vi "Graph with cursors Facade.vi"(0 "Data In":T4, 2 "Display State In":T2, 3 "Container State":T3) -> (6 "Data Out":T4, 7 "Display State Out":T2, 8 "Action":T1)   [LabVIEW 2014, in "Graph with cursors XControl.xctl"]
uses:
  Graph with cursors XControl.xctl
  Graph with cursors Data.ctl
  <vilib>/_xctls/Container State.ctl
  Graph with cursors State.ctl
  <vilib>/_xctls/Action.ctl
  <vilib>/_xctls/XControlSupport.lvlib
panel:
  in  "SaveCursors":bool
  in  "CursorPath":path
  in  "LoadCursors":bool
  in  "Prefix":string
  in  "Save":bool
  in  "Cursor pairs":u32=1 min=1
  out "Graph":waveform(dbl)(graph)
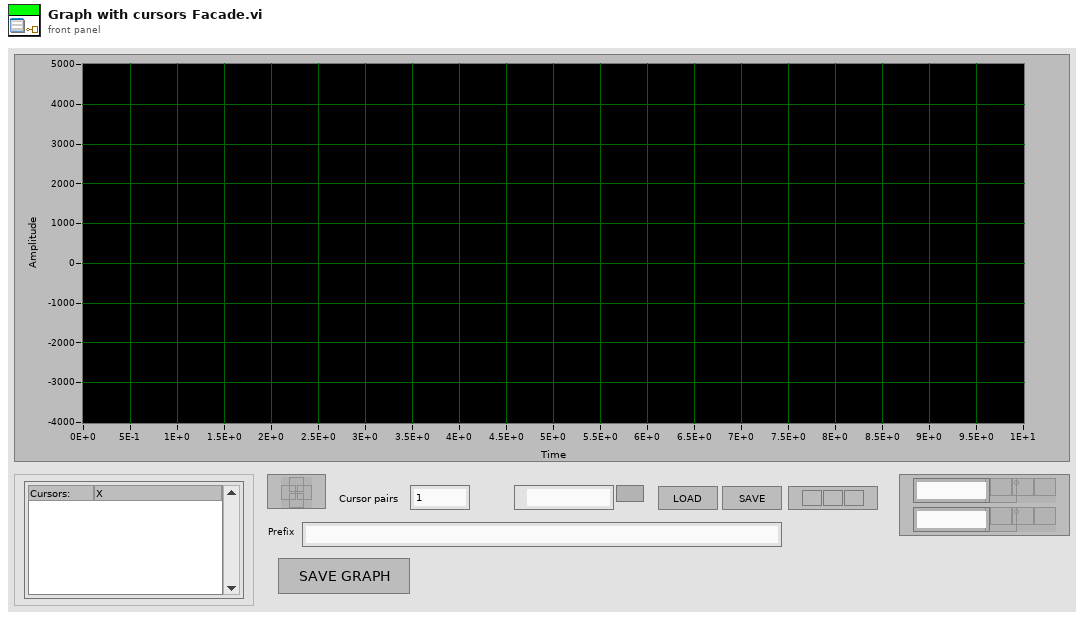
[diagram p1: front panel]
types:
  T1 = typedef "XControlSupport.lvlib/Action.ctl" = cluster{"Data Changed?":bool, "State Changed?":bool, "Action Name":string}
  T2 = typedef "Graph with cursors XControl.xctl/Graph with cursors State.ctl" = cluster{"Cursor names":string[], "Cursor positions":dbl[], "Cursor pairs":i32, "Graph":refnum<vi>, "Prefix":string, "Base path":path}
  T3 = typedef "XControlSupport.lvlib/Container State.ctl" = cluster{"Indicator?":bool, "Run Mode?":bool, " Refnum":refnum<vi>}
  T4 = typedef "Graph with cursors XControl.xctl/Graph with cursors Data.ctl" = waveform(dbl)
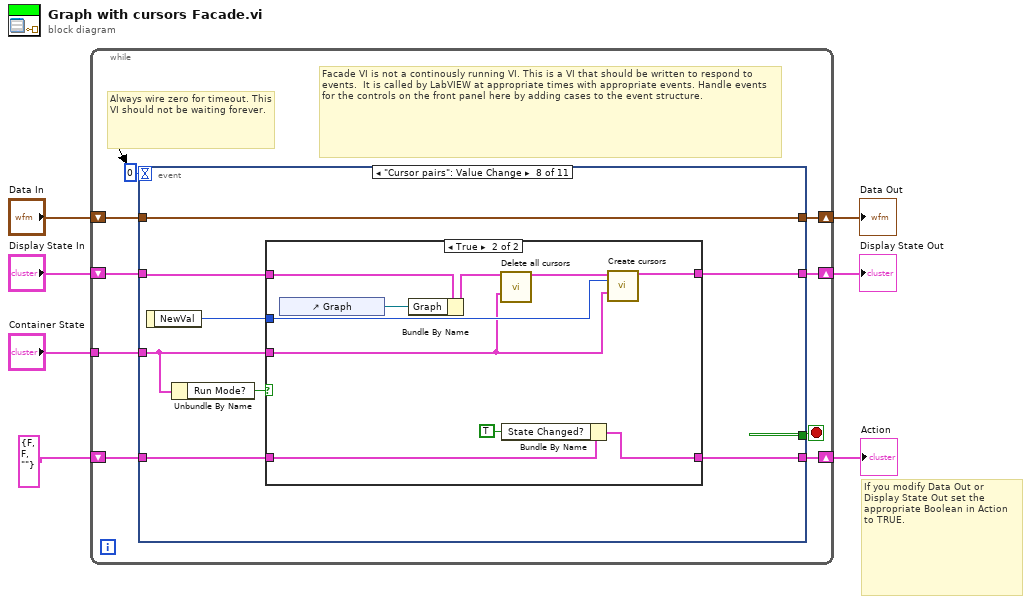
[diagram p0: block diagram]
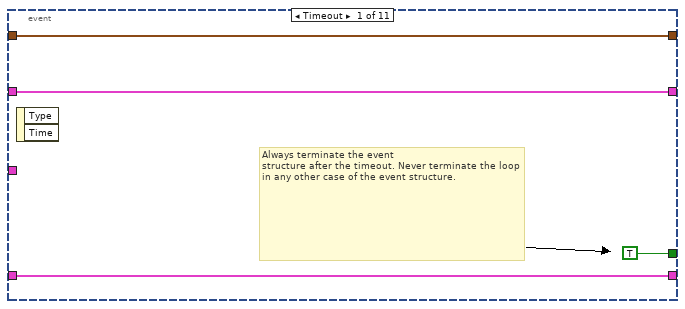
[diagram p2: hidden frame]
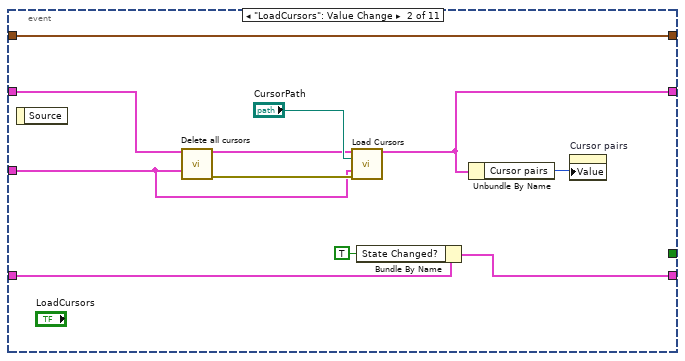
[diagram p3: hidden frame]
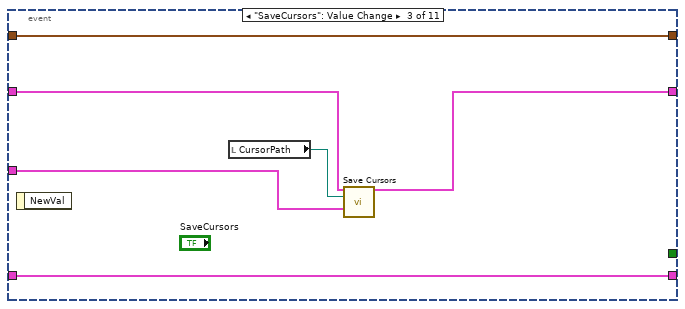
[diagram p4: hidden frame]
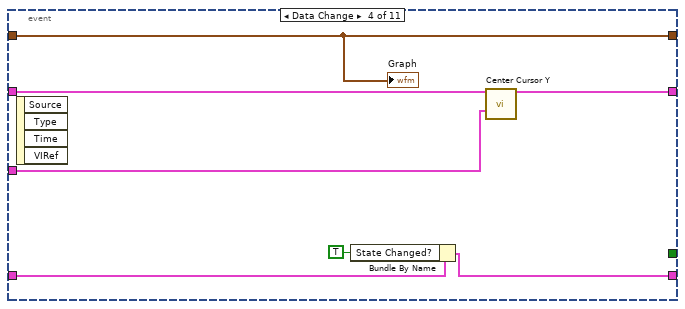
[diagram p5: hidden frame]
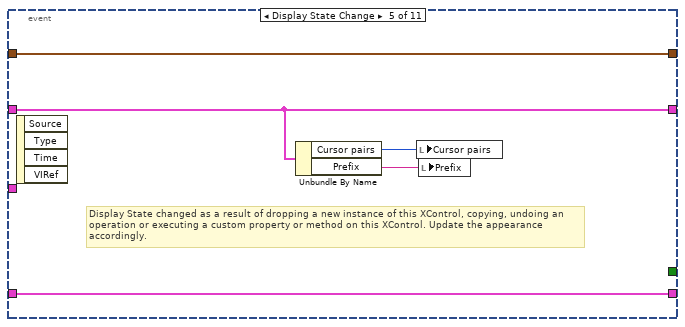
[diagram p6: hidden frame]
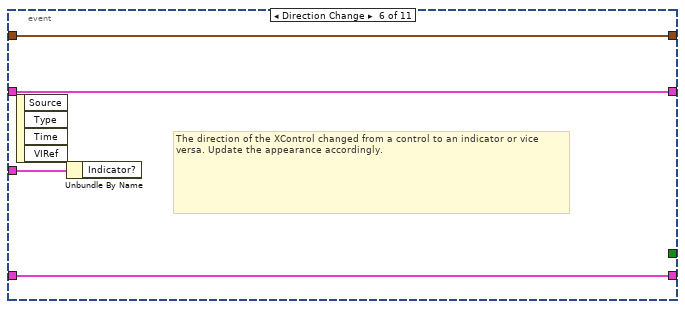
[diagram p7: hidden frame]
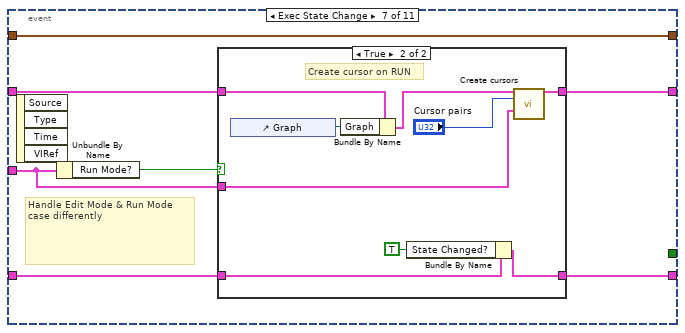
[diagram p8: hidden frame]
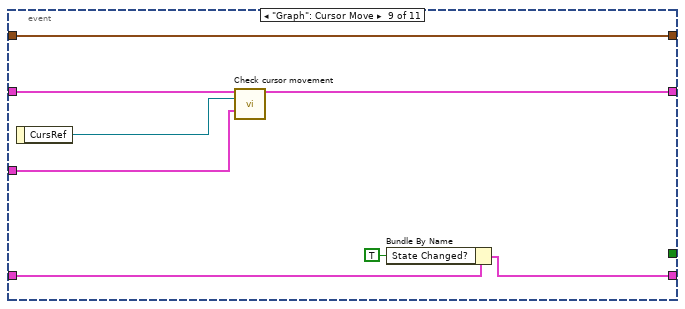
[diagram p11: hidden frame]
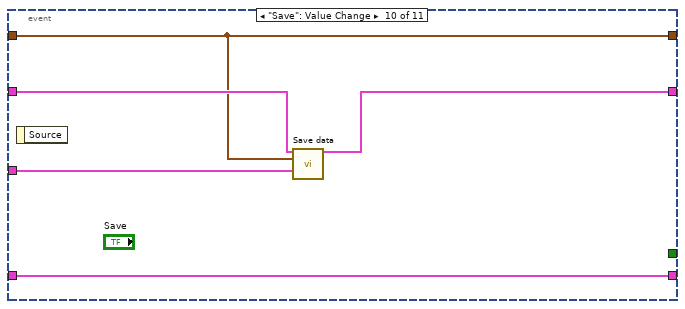
[diagram p12: hidden frame]
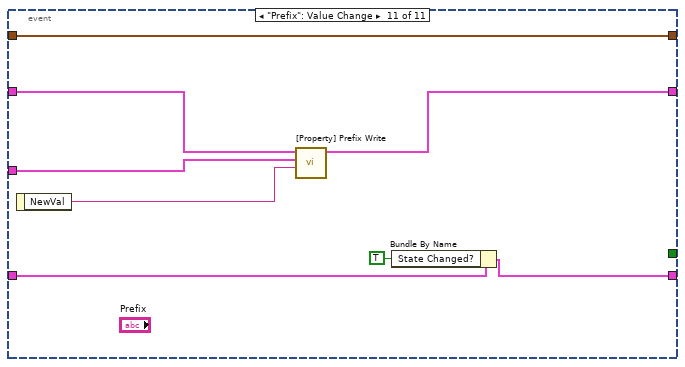
[diagram p13: hidden frame]
diagram:
  # "If you modify Data Out or\nDisplay State Out set the\nappropriate Boolean in Action\nto TRUE."
  n1 = while {
    shift-right: [w15] -> w4
    shift-left: "Display State In" -> [w16]
    tunnel: "Container State" -> [w12]
    shift-right: [w10] -> w7
    shift-left: "Data In" -> [w11]
    shift-right: [w8] -> w3
    shift-left: T1 {"Data Changed?"=FALSE, "State Changed?"=FALSE, "Action Name"=""} ("Action") -> [w9]
    stop <- w14 stop-if-true
    # "Facade VI is not a continously running VI. This is a VI that should be written to respond to events.  It is called by LabVIEW at appropriate times with appropriate events. Handle events for the controls on the front panel here by adding cases to the event structure."
    # "Always wire zero for timeout. This\nVI should not be waiting forever."
    n2 = event shown="[7] \"Cursor pairs\": Value Change" {
      selector: _ -> [_ _ _ _ _ _ _ _ _ _ _]
      dyn-events: _ -> [_ _ _ _ _ _ _ _ _ _ _]
      timeout: 0 -> [_ _ _ _ _ _ _ _ _ _ _]
      tunnel: w16 -> [w18 w23 w34 w42 w47 w52 w59 w76 w98 w103 w108]
      tunnel: [w18 w22 w33 w43 w47 w52 w57 w78 w97 w102 w107] -> w15
      tunnel: [TRUE _ _ _ _ _ _ _ _ _ _] -> w14
      tunnel: w12 -> [_ w24 w32 w38 _ w53 w54 w73 w96 w101 w106]
      tunnel: w11 -> [w17 w31 w37 w44 w49 w51 w60 w79 w99 w100 w112]
      tunnel: [w17 w31 w37 w44 w49 w51 w60 w79 w99 w100 w112] -> w10
      tunnel: [w19 w27 w36 w39 w48 w50 w56 w74 w94 w104 w110] -> w8
      tunnel: w9 -> [w19 w28 w36 w41 w48 w50 w55 w75 w93 w104 w111]
      event Timeout {
        # "Always terminate the event\nstructure after the timeout. Never terminate the loop in any other case of the event structure."
        n3 = event-data() -> ()  [unwired: 1 in, 2 out]
      }
      event "LoadCursors": Value Change {
        n4 = event-data() -> ()  [unwired: 1 in, 1 out]
        n5 = call "Delete all cursors.vi"("Display State In"=w23, "Container State"=w24) -> ("Display State Out"=w26:T2, "error out"=w25:errorcluster)  [unwired: 12 in]
        n6 = call "Load Cursors.vi"("Display State In"=w26, "Path"="CursorPath", "Container State"=w24, "error in (no error)"=w25) -> ("Display State Out"=w22:T2)  [unwired: 10 in, 1 out]
        n7 = Bundle By Name(cluster=w28, "State Changed?"=TRUE) -> (w27:T1)
        n8 = Unbundle By Name(w22) -> ("Cursor pairs"=w21:i32)
        n9 = property on="Cursor pairs" class="DigNum (strict)"("Value"=w21) -> ()  [unwired: 2 in, 2 out]
      }
      event "SaveCursors": Value Change {
        n10 = event-data() -> ()  [unwired: 1 in, 1 out]
        n11 = local read "CursorPath"() -> (w35:path)
        n12 = call "Save Cursors.vi"("Display State In"=w34, "Path"=w35, "Container State"=w32) -> ("Display State Out"=w33:T2)  [unwired: 11 in, 1 out]
      }
      event Data Change {
        n13 = event-data() -> ()  [unwired: 1 in, 4 out]
        n14 = Bundle By Name(cluster=w41, "State Changed?"=TRUE) -> (w39:T1)
        n15 = call "Center Cursor Y.vi"("Display State In"=w42, "Container State"=w38) -> ("Display State Out"=w43:T2)  [unwired: 12 in, 1 out]
        "Graph" <- w44
      }
      event Display State Change {
        # "Display State changed as a result of dropping a new instance of this XControl, copying, undoing an operation or executing a custom property or method on this XControl. Update the appearance accordingly."
        n16 = event-data() -> ()  [unwired: 1 in, 4 out]
        n17 = Unbundle By Name(w47) -> ("Cursor pairs"=w46:i32, "Prefix"=w45:string)
        n18 = local write "Cursor pairs"(w46) -> ()
        n19 = local write "Prefix"(w45) -> ()
      }
      event Direction Change {
        # "The direction of the XControl changed from a control to an indicator or vice versa. Update the appearance accordingly."
        n20 = event-data() -> ()  [unwired: 1 in, 4 out]
        n21 = Unbundle By Name(w53) -> ()  [unwired: 1 out]
      }
      event Exec State Change {
        # "Handle Edit Mode & Run Mode\ncase differently"
        n22 = event-data() -> ()  [unwired: 1 in, 4 out]
        n23 = Unbundle By Name(w54) -> ("Run Mode?"=w58:bool)
        n24 = case shown="True" w58 {
          tunnel: w59 -> [w62 w70]
          tunnel: [w62 w69] -> w57
          tunnel: [w61 w65] -> w56
          tunnel: w55 -> [w61 w66]
          tunnel: w54 -> [_ w67]
          frame False {
          }
          frame True {
            # "Create cursor on RUN"
            n25 = control-ref of="Graph"() -> (w71:refnum<vi>)
            n26 = Bundle By Name(cluster=w70, "Graph"=w71) -> (w68:T2)
            n27 = Bundle By Name(cluster=w66, "State Changed?"=TRUE) -> (w65:T1)
            n28 = call "Create cursors.vi"("Display State In"=w68, "Cursor pairs"="Cursor pairs", "Container State"=w67) -> ("Display State Out"=w69:T2)  [unwired: 11 in, 1 out]
          }
        }
      }
      event "Cursor pairs": Value Change {
        n29 = event-data() -> ("NewVal"=w77:u32)  [unwired: 1 in]
        n30 = Unbundle By Name(w73) -> ("Run Mode?"=w72:bool)
        n31 = case shown="True" w72 {
          tunnel: [w81 w91] -> w78
          tunnel: w77 -> [_ w90]
          tunnel: w73 -> [_ w88]
          tunnel: w76 -> [w81 w84]
          tunnel: w75 -> [w80 w86]
          tunnel: [w80 w85] -> w74
          frame False {
          }
          frame True {
            n32 = control-ref of="Graph"() -> (w82:refnum<vi>)
            n33 = Bundle By Name(cluster=w84, "Graph"=w82) -> (w83:T2)
            n34 = call "Delete all cursors.vi"("Display State In"=w83, "Container State"=w88) -> ("Display State Out"=w89:T2)  [unwired: 12 in, 1 out]
            n35 = Bundle By Name(cluster=w86, "State Changed?"=TRUE) -> (w85:T1)
            n36 = call "Create cursors.vi"("Display State In"=w89, "Cursor pairs"=w90, "Container State"=w88) -> ("Display State Out"=w91:T2)  [unwired: 11 in, 1 out]
          }
        }
      }
      event "Graph": Cursor Move {
        n37 = event-data() -> ("CursRef"=w95:refnum<vi>)  [unwired: 1 in]
        n38 = call "Check cursor movement.vi"("Display State In"=w98, "CursRef"=w95, "Container State"=w96) -> ("Display State Out"=w97:T2)  [unwired: 11 in, 1 out]
        n39 = Bundle By Name(cluster=w93, "State Changed?"=TRUE) -> (w94:T1)
      }
      event "Save": Value Change {
        n40 = event-data() -> ()  [unwired: 1 in, 1 out]
        n41 = call "Save data.vi"("Display State In"=w103, "Data"=w100, "Container State"=w101) -> ("Display State Out"=w102:T2)  [unwired: 11 in, 1 out]
      }
      event "Prefix": Value Change {
        n42 = event-data() -> ("NewVal"=w105:string)  [unwired: 1 in]
        n43 = call "[Property] Prefix Write.vi"("Value"=w105, "Container State"=w106, "Display State In"=w108) -> ("Display State Out"=w107:T2)  [unwired: 3 in, 1 out]
        n44 = Bundle By Name(cluster=w111, "State Changed?"=TRUE) -> (w110:T1)
      }
    }
  }
  "Display State Out" <- w4
  "Data Out" <- w7
  "Action" <- w3
